vi "DeQueue.vi"(8 "ErrorArray":errorcluster[](array[cluster])) -> (0 "ErrorArray":errorcluster[](array[cluster]), 1 "Data":variant, 2 "Message":string)   [LabVIEW 2014, in "TestBase.lvclass"]
uses:
  TestBase.lvclass
  clQueMsgType.ctl
  <vilib>/Utility/error.llb/Error Cluster From Error Code.vi
  <vilib>/ErrorRing/Error Ring.xnode
  <userlib>/NIST/NISTErrorLib/NISTErrorLib.lvlib
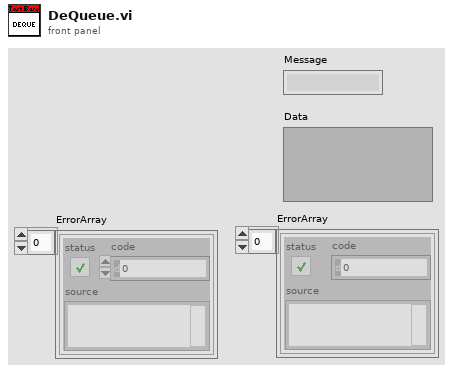
[diagram p1: front panel]
types:
  T1 = typedef "TestBase.lvclass/clQueMsgType.ctl" = cluster{"Message":string, "Data":variant}
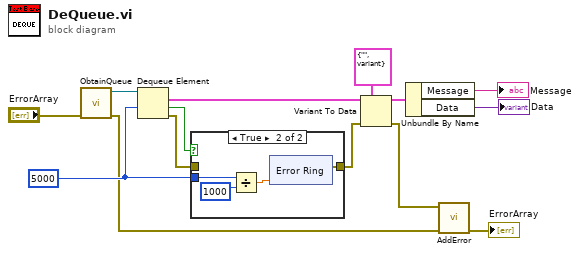
[diagram p0: block diagram]
diagram:
  w11 = 5000 ("timeout in ms (-1)")
  n1 = call "ObtainQueue.vi"("ErrorArray"="ErrorArray") -> ("ErrorArray."=w8:errorcluster[], "TstQue"=w13:refnum<queue>)  [unwired: 9 in]
  n2 = Dequeue Element(queue=w13, timeout in ms (-1)=w11) -> (element=w7:T1, timed out?=w12:bool, error out=w10:errorcluster)  [unwired: 1 in, 1 out]
  n3 = case shown="True" w12 {
    tunnel: w11 -> [_ w19]
    tunnel: [w15 w16] -> w2
    tunnel: w10 -> [w15 _]
    frame False {
    }
    frame True {
      n4 = Divide(x=w19, y=1000) -> (x/y=w17:dbl)
      n5 = xnode "Error Ring"("parameter 0"=w17) -> ("error out"=w16:errorcluster)
    }
  }
  n6 = Variant To Data(error in=w2, type=T1 {"Message"="", "Data"=variant} ("clQueMsgType"), Variant=w7) -> (data=w5:T1, error out=w1:errorcluster)
  n7 = Unbundle By Name(w5) -> ("Message"=→"Message":string, "Data"=→"Data":variant)
  n8 = call <userlib>:"AddError.vi"("ErrorArray"=w8, "error in (no error)"=w1) -> ("ErrorArray"=→"ErrorArray":errorcluster[])  [unwired: 8 in, 1 out]
